vi "Notify Subscribers.vi"(8 "error in (no error)":errorcluster, 10 "PublishRequest":refnum<class "PublishRequest.lvclass">, 11 "Topic in":refnum<class "Topic.lvclass">) -> (0 "error out":errorcluster, 3 "Topic out":refnum<class "Topic.lvclass">)   [LabVIEW 2018, in "MVA Framework.lvlib" / "Mediator.lvlib" / "Topic.lvclass"]
doc: "通知订阅者"
uses:
  Topic.lvclass
  IMediator/PublishRequest/PublishRequest.lvclass
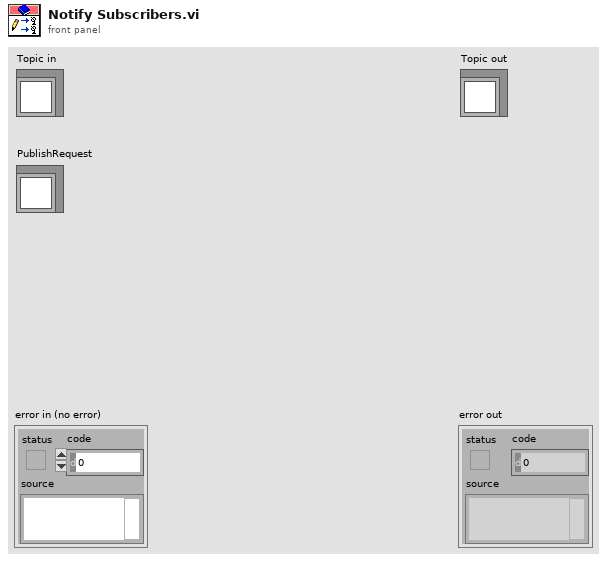
[diagram p1: front panel]
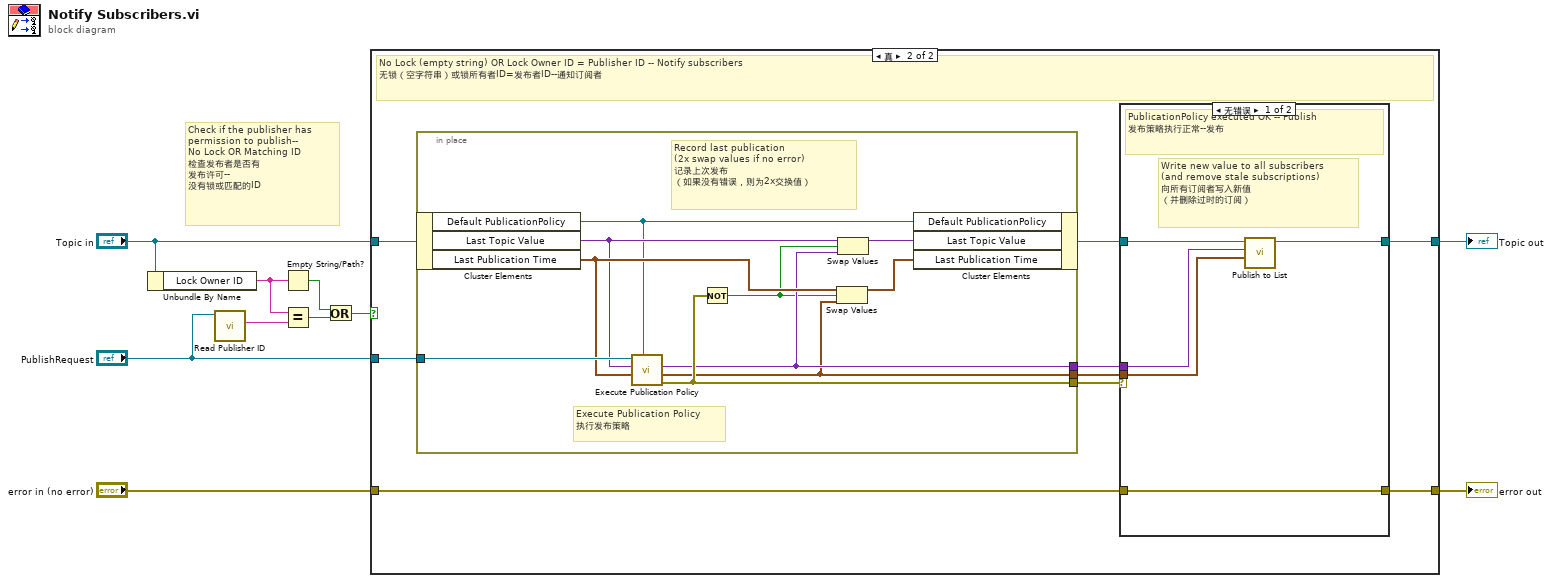
[diagram p0: block diagram]
diagram:
  # "Check if the publisher has\npermission to publish--\nNo Lock OR Matching ID\n检查发布者是否有\n发布许可--\n没有锁或匹配的ID"
  n1 = Unbundle By Name("Topic in") -> ("Lock Owner ID"=w6:string)
  n2 = call "Read Publisher ID.vi"("PublishRequest In"="PublishRequest") -> ("Publisher ID"=w1:string)  [unwired: 10 in]
  n3 = Empty String/Path?(string/path=w6) -> (empty?=w5:bool)
  n4 = Equal?(x=w6, y=w1) -> (x = y?=w4:bool)
  n5 = Or(x=w5, y=w4) -> (x .or. y?=w3:bool)
  n6 = case shown="真" w3 {
    tunnel: "error in (no error)" -> [w12 w21]
    tunnel: [w12 w20] -> w9
    tunnel: [w11 w19] -> w8
    tunnel: "Topic in" -> [w11 w14]
    tunnel: "PublishRequest" -> [_ w18]
    frame False {
      # "This publication was not from the lock holder -- Ignore it\n此出版物不是来自锁夹的--忽略它"
    }
    frame True {
      # "No Lock (empty string) OR Lock Owner ID = Publisher ID -- Notify subscribers\n无锁（空字符串）或锁所有者ID=发布者ID--通知订阅者"
      n7 = in-place {
        in-place-border: w18 -> [w31]
        in-place-border: [w24] -> w17
        in-place-border: [w27] -> w16
        in-place-border: [w22] -> w15
        # "Record last publication\n(2x swap values if no error)\n记录上次发布\n（如果没有错误，则为2x交换值）"
        # "Execute Publication Policy\n执行发布策略"
        n8 = in-place-cluster #1(w14) -> ("Default PublicationPolicy"=w25:refnum<class "IPublicationPolicy.lvclass">, "Last Topic Value"=w26:variant, "Last Publication Time"=w29:timestamp)
        n9 = call-dynamic "Execute Publication Policy.vi"("Default PublicationPolicy"=w25, "Last Publish Time"=w29, "Last Published Value"=w26, "PublishRequest"=w31) -> ("error out (Reject Publication)"=w27:errorcluster, "Publication Time"=w22:timestamp, "Value to Publish"=w24:variant)  [unwired: 5 in]
        n10 = Not(x=w27) -> (.not. x?=w23:bool)
        n11 = Swap Values(12:w29, 13:w23, 14:w22) -> (1:w28:timestamp)  [unwired: 1 out]
        n12 = Swap Values(12:w26, 13:w23, 14:w24) -> (1:w30:variant)  [unwired: 1 out]
        n13 = in-place-cluster #1("Default PublicationPolicy"=w25, "Last Topic Value"=w30, "Last Publication Time"=w28) -> (w13:refnum<class "Topic.lvclass">)
      }
      n14 = case shown="无错误" w16 {
        tunnel: w21 -> [w36 w38]
        tunnel: [w36 w38] -> w20
        tunnel: [w35 w37] -> w19
        tunnel: w13 -> [w34 w37]
        tunnel: w17 -> [w32 _]
        tunnel: w15 -> [w33 _]
        frame No Error {
          # "Write new value to all subscribers\n(and remove stale subscriptions)\n向所有订阅者写入新值\n（并删除过时的订阅）"
          # "PublicationPolicy executed OK -- Publish\n发布策略执行正常--发布"
          n15 = call "Publish to List.vi"("Publication Time"=w33, "Value to Publish"=w32, "Topic in"=w34) -> ("Topic out"=w35:refnum<class "Topic.lvclass">)  [unwired: 8 in]
        }
        frame Error {
          # "Error executing PublicationPolicy -- Do not publish"
        }
      }
    }
  }
  "error out" <- w9
  "Topic out" <- w8
